vi "Renishaw-XL80_GetEC10Version.vi"(8 "error in (no error)":errorcluster, 11 "Renishaw-XL80_EMU in":refnum<class "Renishaw-XL80_EMU.lvclass">) -> (0 "error out":errorcluster, 2 "EC10Version":string, 3 "Renishaw-XL80_EMU out":refnum<class "Renishaw-XL80_EMU.lvclass">)   [LabVIEW 2024, in "Renishaw-XL80_EMU.lvclass"]
doc: "This read only property returns the version string of the EC10.\n\nDefinition\nHRESULTget_EC10Version( [out, retval] BSTR* pVal);\nParameters\npVal\nA variable that will be set to the version string of the EC10.\n\nComments\nThis property will return with an HRESULT of E_FAIL if the client has not previously connected to a DX10 by calling Connect.\n\nThe property will normally return an HRESULT of S_OK. However, it will return E_POINTER if the client supplies a null pointer for pVal, and in extremely low memory conditions it will return E_NOMEMORY.\n\nNote: if there is a XL laser connected to the DX10Adaptor COM interface this property will return the firmare version of the associated XC compensator."
uses:
  Renishaw-XL80_EMU.lvclass
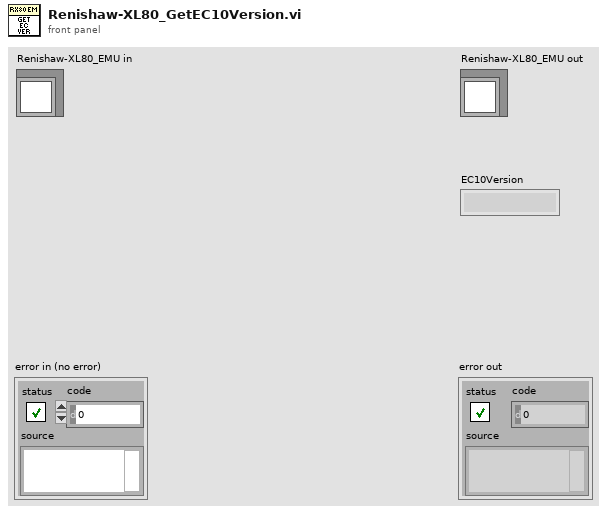
[diagram p1: front panel]
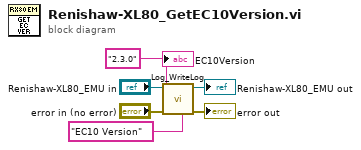
[diagram p0: block diagram]
diagram:
  w1 = "2.3.0" ("Additional text")
  n1 = call-dynamic "Log_WriteLog.vi"("Additional text"="EC10 Version", "error in (no error)"="error in (no error)", "Response"=w1, "Log in"="Renishaw-XL80_EMU in") -> ("error out"=→"error out":errorcluster, "Log out"=→"Renishaw-XL80_EMU out":refnum<class "Renishaw-XL80_EMU.lvclass">)  [unwired: 6 in]
  "EC10Version" <- w1
